vi "testBenchmarkSystemDefinitionFails.vi"(8 "error in (no error)":errorcluster, 11 "TestCase in":refnum<class "VeriStandTestCaseSystemTests.lvclass">) -> (0 "error out":errorcluster, 3 "TestCase out":refnum<class "VeriStandTestCaseSystemTests.lvclass">)   [LabVIEW 2027, in "VeriStandTestCaseSystemTests.lvclass"]
uses:
  VeriStandTestCaseSystemTests.lvclass
  Source/VeriStandTestCase/VeriStandTestCase.lvclass
  C:/Program Files/National Instruments/LabVIEW 2027/vi.lib/addons/_JKI Toolkits/VI Tester/TestCase.llb/TestCase.lvclass
  <vilib>/addons/_JKI Toolkits/VI Tester/TestCase.llb/TestCase.lvclass
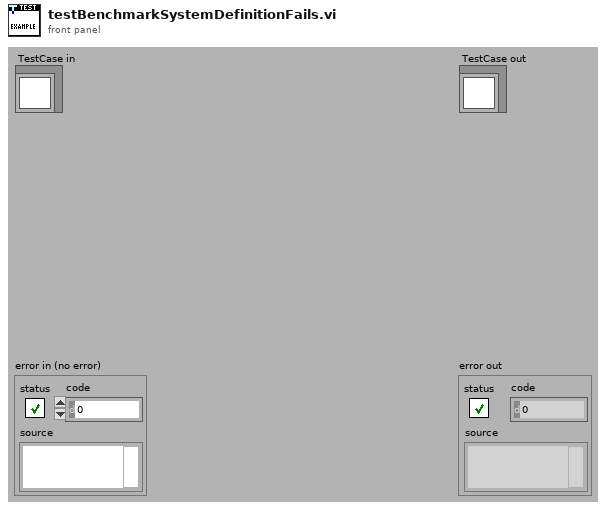
[diagram p1: front panel]
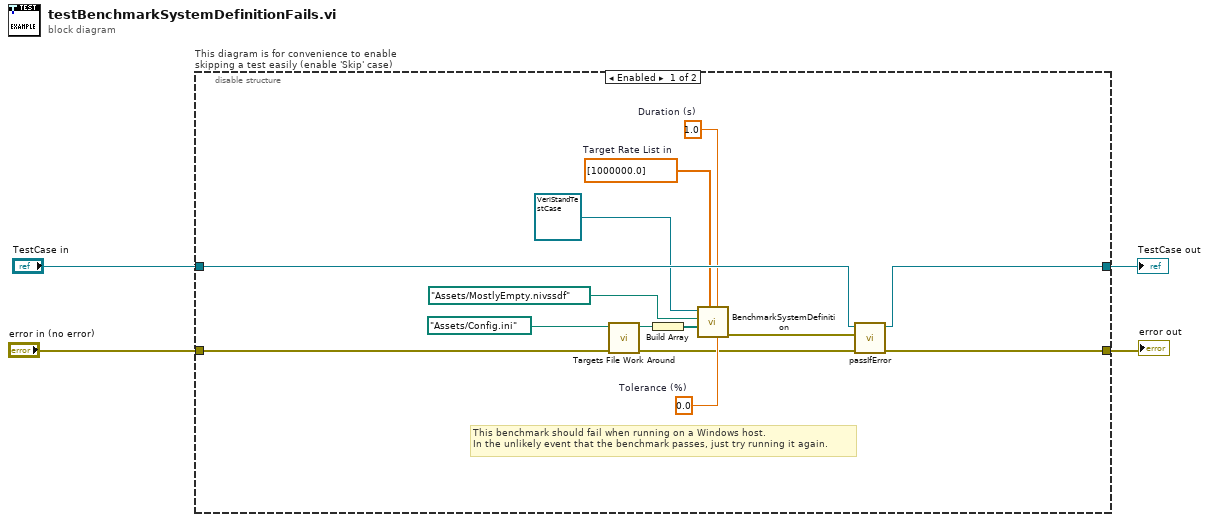
[diagram p0: block diagram]
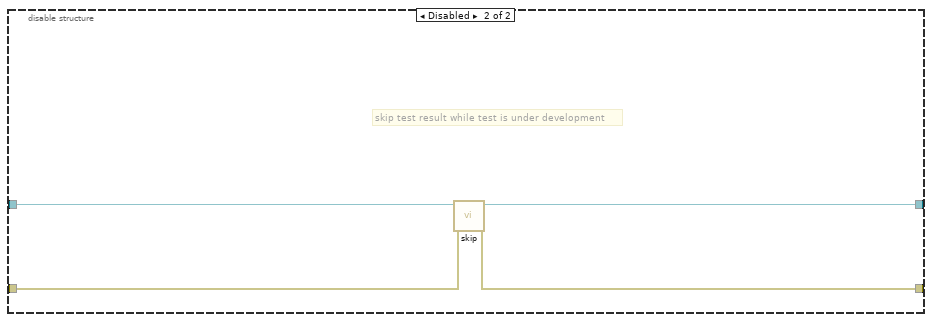
[diagram p2: hidden frame]
diagram:
  n1 = disable-structure "This diagram is for convenience to enable skipping a test easily (enable 'Skip' case)" shown="Enabled" {
    disable-tunnel: "TestCase in" -> [w16 w22]
    disable-tunnel: [w15 w20] -> w1
    disable-tunnel: [w17 w21] -> w3
    disable-tunnel: "error in (no error)" -> [w18 w19]
    frame Enabled {
      w9 = 0.0  # Tolerance (%)
      w10 = 1.0  # Duration (s)
      w11 = dbl[] [1000000.0]  # Target Rate List in
      # "This benchmark should fail when running on a Windows host.\nIn the unlikely event that the benchmark passes, just try running it again."
      n2 = call "Targets File Work Around.vi"("error in (no error)"=w18, "overrides file in"=path "Assets/Config.ini" ("overrides files")) -> ("error out"=w8:errorcluster, "overrides file out"=w6:path)  [unwired: 8 in]
      n3 = Build Array(w6) -> (w5:path[])
      n4 = call-dynamic "BenchmarkSystemDefinition.vi"("Tolerance (%)"=w9, "Duration (s)"=w10, "Target Rate List in"=w11, "overrides files"=w5, "System Definition File"=path "Assets/MostlyEmpty.nivssdf", "VeriStandTestCase in"=refnum<class "VeriStandTestCase.lvclass"> refnum ("VeriStand Test Case in")) -> ("error out"=w14:errorcluster)  [unwired: 4 in, 1 out]
      n5 = call-dynamic "passIfError.vi"("error in (no error)"=w8, "error"=w14, "TestCase in"=w16) -> ("error out"=w17:errorcluster, "TestCase out"=w15:refnum<class "VeriStandTestCaseSystemTests.lvclass">)  [unwired: 7 in]
    }
    frame Disabled {
      # "skip test result while test is under development"
      n6 = call <vilib>:"skip.vi"("error in (no error)"=w19, "TestCase in"=w22) -> ("error out"=w21:errorcluster, "TestCase out"=w20:refnum<class "VeriStandTestCaseSystemTests.lvclass">)  [unwired: 8 in]
    }
  }
  "error out" <- w3
  "TestCase out" <- w1
